vi "AlazarSetExternalTrigger.vi"(3 "error in (no error)":errorcluster, 4 "Range ID":u32(ring) items=["5 V", "1 V", "TTL"], 5 "Coupling ID":u32(ring)=2 items=["AC"=1, "DC"=2], 6 "Handle":u64) -> (0 "error out":errorcluster, 1 "Return Code":u32, 2 "Handle":u64)   [LabVIEW 2018]
doc: "Set the external trigger range and coupling."
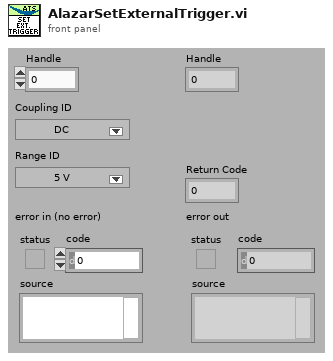
[diagram p1: front panel]
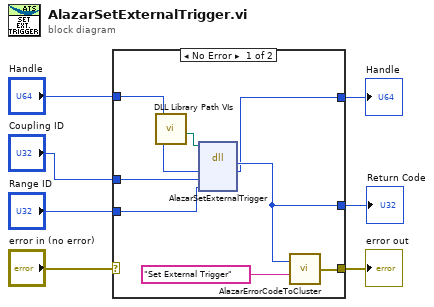
[diagram p0: block diagram]
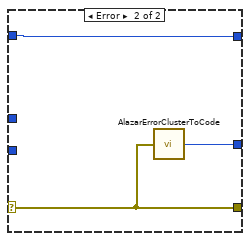
[diagram p2: hidden frame]
diagram:
  n1 = case shown="No Error" "error in (no error)" {
    selector: "error in (no error)" -> [_ w18]
    tunnel: [w12 w18] -> w6
    tunnel: [w14 w17] -> w5
    tunnel: "Handle" -> [w15 w16]
    tunnel: [w11 w16] -> w4
    tunnel: "Coupling ID" -> [w10 _]
    tunnel: "Range ID" -> [w9 _]
    frame No Error {
      n2 = call "DLL Library Path VIs.vi"() -> ("Alazar"=w8:path)  [unwired: 8 in, 3 out]
      n3 = dll-call lib="C:/Project/SerialSectOCT - FFT GPU/SerialSectOCT/Labview Software/DLL/ATSApi.dll" fn="AlazarSetExternalTrigger"(path in=w8, "handle"=w15, "coupling"=w10, "range"=w9) -> ("return type"=w14:u32, "handle"=w11:u64)  [unwired: 4 in, 2 out]
      n4 = call "AlazarErrorCodeToCluster.vi"("Message"="Set External Trigger", "Error Code"=w14) -> ("error out"=w12:errorcluster)
    }
    frame Error {
      n5 = call "AlazarErrorClusterToCode.vi"("error in (no error)"=w18) -> ("Error Code"=w17:u32)
    }
  }
  "Handle" <- w4
  "error out" <- w6
  "Return Code" <- w5
